vi "MAC Address Fetcher_2016.vi"(8 "error in (no error)":errorcluster) -> (0 "error out":errorcluster, 3 "MAC Addresses":string[](array[string]))   [LabVIEW 2016]
doc: "This VI calls a Windows shell command that fetches details of the installed Network Interface Cards. It then searches for valid Physical (MAC) Addresses and populates an array. If \"All adapters\" is set to True, then the whole array will be output. otherwise, only the first element will be output, which should correspond to the primary ethernet adapter."
uses:
  <vilib>/regexp/Match Regular Expression.xnode
panel:
  out "Adapter type":string[](array[string])
  out "Shell Output":string
  # "Network card MAC Address Fetcher"
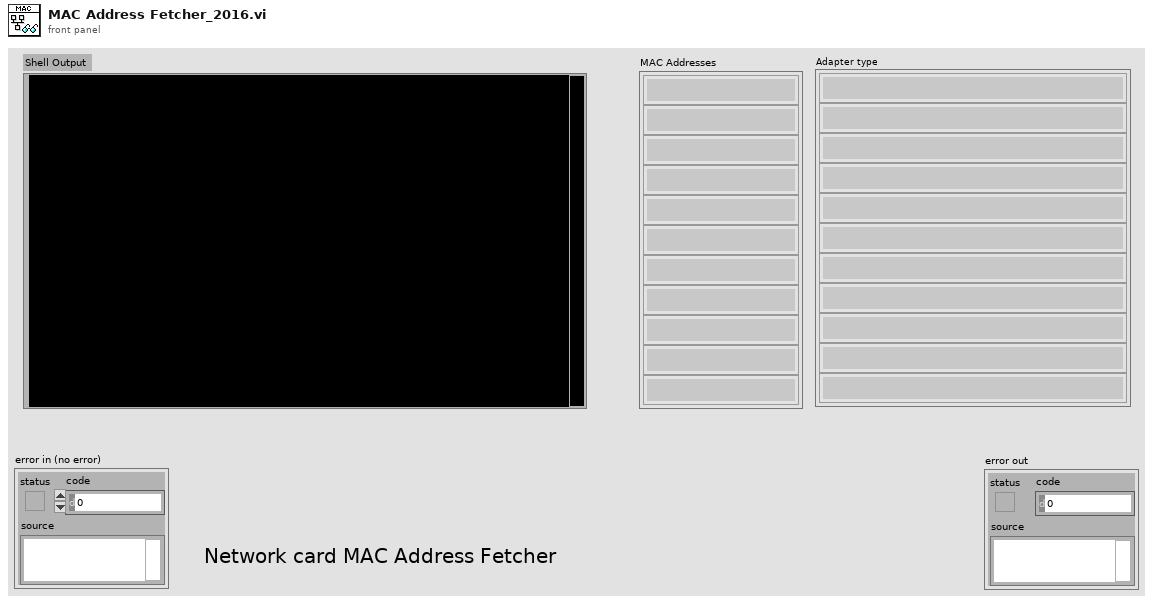
[diagram p1: front panel]
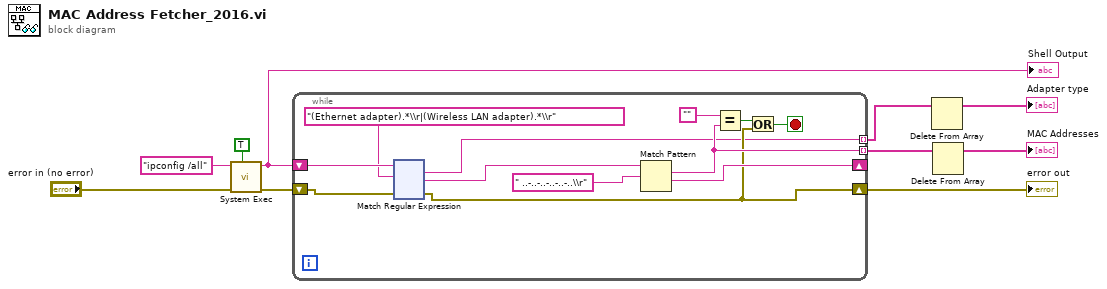
[diagram p0: block diagram]
diagram:
  n1 = call <vilib>:"System Exec.vi"("run minimized? (F)"=TRUE, "error in (no error)"="error in (no error)", "command line"="ipconfig /all") -> ("error out"=w6:errorcluster, "standard output"=w3:string)  [unwired: 5 in, 2 out]
  "Shell Output" <- w3
  n2 = while {
    shift-right: [w21] -> _
    shift-left: w3 -> [w16]
    tunnel: [w20] -> w8 mode=indexing
    shift-right: [w14] -> w5
    shift-left: w6 -> [w15]
    tunnel: [w11] -> w2 mode=indexing
    stop <- w17 stop-if-true
    n3 = xnode "Match Regular Expression"("input string"=w16, "regular expression"="(Ethernet adapter).*\\r|(Wireless LAN adapter).*\\r", "error in"=w15) -> ("whole match"=w11:string, "after match"=w12:string, "error out"=w14:errorcluster)  [unwired: 3 in, 2 out]
    n4 = Match Pattern(string=w12, regular expression=" ..-..-..-..-..-..\\r") -> (match substring=w20:string, after substring=w21:string)  [unwired: 1 in, 2 out]
    n5 = Equal?(x="", y=w20) -> (x = y?=w18:bool)
    n6 = Or(x=w18, y=w14) -> (x .or. y?=w17:bool)
  }
  "error out" <- w5
  n7 = Delete From Array(array=w2) -> (array with subset deleted=→"Adapter type":string[])  [unwired: 2 in, 1 out]
  n8 = Delete From Array(array=w8) -> (array with subset deleted=→"MAC Addresses":string[])  [unwired: 2 in, 1 out]
